vi "GenerateTriggeredStimulus.vi"(8 "error in (no error)":errorcluster, 11 "Stimulus in":refnum<class "FullWormRailsTriggeredBySmallEllipseRatio.lvclass">) -> (0 "error out":errorcluster, 2 "TriggeredStimulus":sgl[][](array[numeric]), 3 "Stimulus out":refnum<class "FullWormRailsTriggeredBySmallEllipseRatio.lvclass">)   [LabVIEW 2019, in "FullWormRailsTriggeredBySmallEllipseRatio.lvclass"]
uses:
  FullWormRailsTriggeredBySmallEllipseRatio.lvclass
  FullWormRailsTriggeredBySmallEllipseRatio.lvclass/FullWormRailsTriggeredBySmallEllipseRatio.ctl
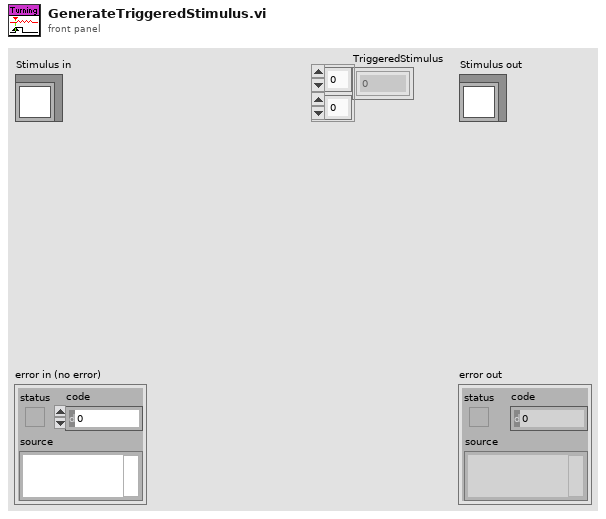
[diagram p1: front panel]
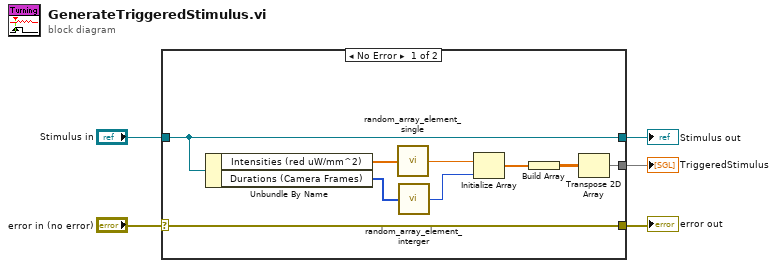
[diagram p0: block diagram]
diagram:
  n1 = case shown="No Error" "error in (no error)" {
    selector: "error in (no error)" -> [w14 w16]
    tunnel: [w14 w16] -> w1
    tunnel: [w13 w15] -> w2
    tunnel: "Stimulus in" -> [w13 w15]
    tunnel: [w6 _] -> w3
    frame No Error {
      n2 = Unbundle By Name(w13) -> ("Intensities (red uW/mm^2)"=w12:sgl[], "Durations (Camera Frames)"=w11:i32[])
      n3 = call "random_array_element_single.vi"("Array of numbers"=w12) -> ("Randomly selected number"=w10:sgl)
      n4 = call "random_array_element_interger.vi"("Array of numbers"=w11) -> ("Randomly selected number"=w9:i32)
      n5 = Initialize Array(w10, w9) -> (w8:sgl[])
      n6 = Build Array(w8) -> (w7:sgl[][])
      n7 = Transpose 2D Array(2D array=w7) -> (transposed array=w6:sgl[][])
    }
    frame Error {
    }
  }
  "error out" <- w1
  "Stimulus out" <- w2
  "TriggeredStimulus" <- w3
